vi "Measure Pulse Guard Pulse Width.vi"(7 "Pulse Phase":enum16{"Stimulus", "Recovery"}(ring), 8 "error in (no error)":errorcluster, 9 "Second Edge Threshold":dbl=4.25, 10 "First Edge Threshold":dbl=5.25, 11 "Input Waveform":waveform(dbl)={"t0"=timestamp(3473263002.422 s since 1904-01-01), "dt"=1e-05, "Y"=[]}) -> (0 "error out":errorcluster, 2 "Pulse Width":dbl)   [LabVIEW 2010]
uses:
  <vilib>/measure/mamon.llb/Waveform Peak Detection for 1 Chan.vi
  <vilib>/measure/NI_MAPro.lvlib
panel:
  out "Waveform in ( graph )":dbl[](graph)
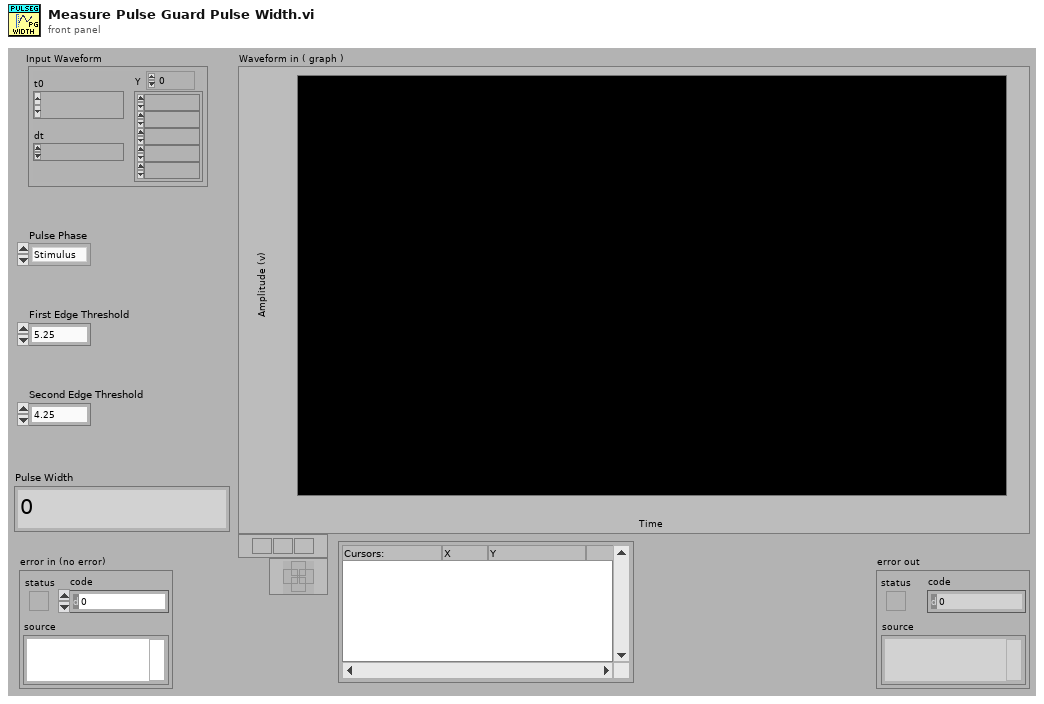
[diagram p1: front panel]
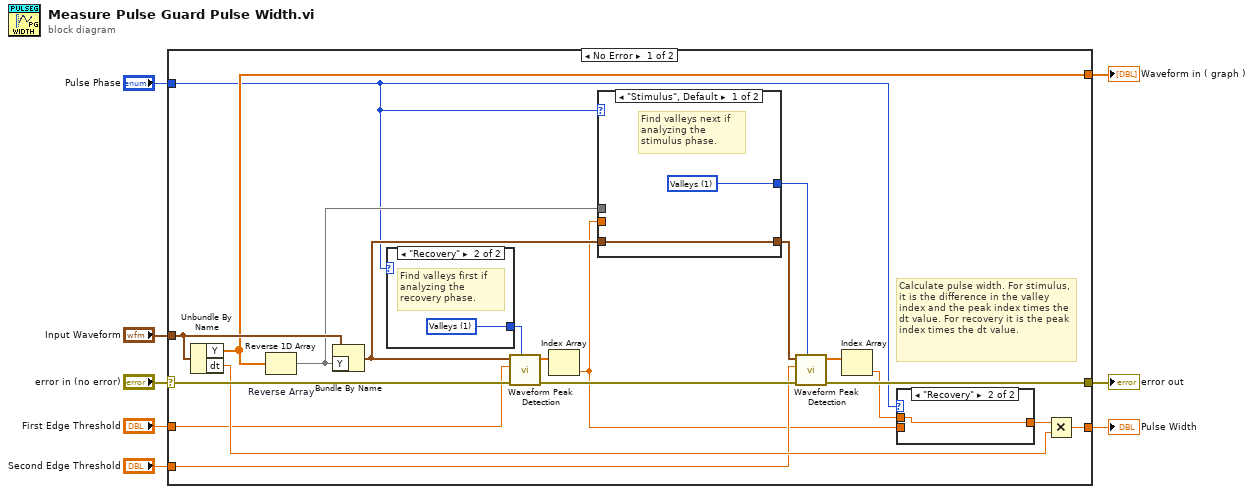
[diagram p0: block diagram]
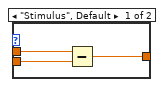
[diagram p2: hidden frame]
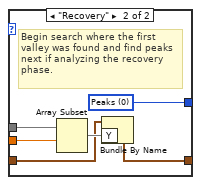
[diagram p3: hidden frame]
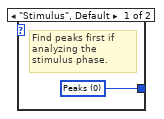
[diagram p4: hidden frame]
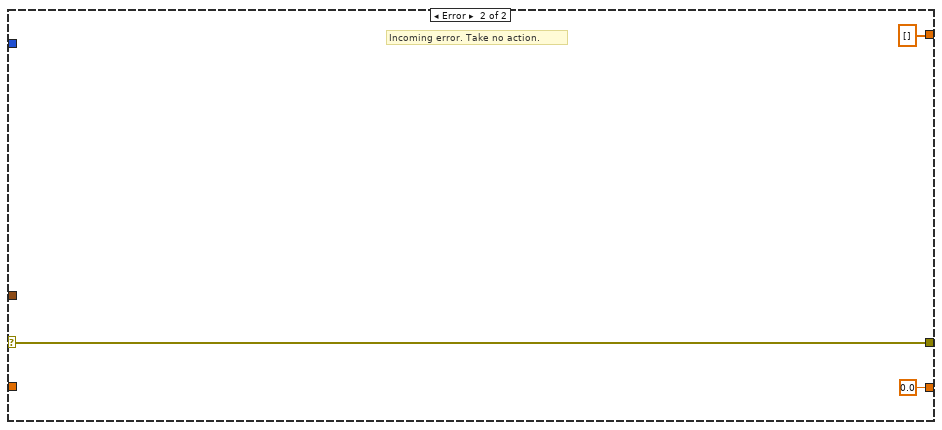
[diagram p5: hidden frame]
diagram:
  n1 = case shown="No Error" "error in (no error)" {
    selector: "error in (no error)" -> [w19 w45]
    tunnel: [w17 0.0] -> w8
    tunnel: [w18 dbl[] [] ("Y")] -> w7
    tunnel: "Second Edge Threshold" -> [w15 _]
    tunnel: "First Edge Threshold" -> [w9 _]
    tunnel: [w26 w45] -> w3
    tunnel: "Input Waveform" -> [w27 _]
    tunnel: "Pulse Phase" -> [w11 _]
    frame No Error {
      # "Calculate pulse width. For stimulus, it is the difference in the valley index and the peak index times the dt value. For recovery it is the peak index times the dt value."
      n2 = Unbundle By Name(w27) -> ("Y"=w18:dbl[], "dt"=w16:dbl)
      n3 = Reverse 1D Array "Reverse Array"(array=w18) -> (reversed array=w14:dbl[])
      n4 = Bundle By Name(cluster=w27, "Y"=w14) -> (w28:waveform(dbl))
      n5 = case shown="\"Recovery\"" w11 {
        tunnel: [w41 w42] -> w24
        frame "Stimulus", Default {
          w41 = u16 0 items=["Peaks", "Valleys"] ("peaks/valleys")
          # "Find peaks first if analyzing the stimulus phase."
        }
        frame "Recovery" {
          w42 = u16 1 items=["Peaks", "Valleys"] ("peaks/valleys")
          # "Find valleys first if analyzing the recovery phase."
        }
      }
      n6 = call-poly <vilib>:"Waveform Peak Detection.vi"("peaks/valleys"=w24, "error in"=w19, "threshold"=w9, "Signal In"=w28) -> ("error out"=w25:errorcluster, "Locations"=w23:dbl[])  [unwired: 3 in, 3 out]
      n7 = Index Array(array=w23) -> (element=w13:dbl)  [unwired: 1 in]
      n8 = case shown="\"Stimulus\", Default" w11 {
        tunnel: w14 -> [_ w40]
        tunnel: w13 -> [_ w39]
        tunnel: w28 -> [w34 w37]
        tunnel: [w34 w36] -> w12
        tunnel: [w33 w35] -> w10
        frame "Stimulus", Default {
          w33 = u16 1 items=["Peaks", "Valleys"] ("peaks/valleys")
          # "Find valleys next if analyzing the stimulus phase."
        }
        frame "Recovery" {
          w35 = u16 0 items=["Peaks", "Valleys"] ("peaks/valleys")
          # "Begin search where the first valley was found and find peaks next if analyzing the recovery phase."
          n9 = Array Subset(array=w40, index=w39) -> (w38:dbl[])  [unwired: 1 in]
          n10 = Bundle By Name(cluster=w37, "Y"=w38) -> (w36:waveform(dbl))
        }
      }
      n11 = call-poly <vilib>:"Waveform Peak Detection.vi"("peaks/valleys"=w10, "error in"=w25, "threshold"=w15, "Signal In"=w12) -> ("error out"=w26:errorcluster, "Locations"=w22:dbl[])  [unwired: 3 in, 3 out]
      n12 = Index Array(array=w22) -> (element=w21:dbl)  [unwired: 1 in]
      n13 = case shown="\"Recovery\"" w11 {
        tunnel: w21 -> [w31 w32]
        tunnel: [w30 w32] -> w20
        tunnel: w13 -> [w29 _]
        frame "Stimulus", Default {
          n14 = Subtract(x=w31, y=w29) -> (x-y=w30:dbl)
        }
        frame "Recovery" {
        }
      }
      n15 = Multiply(x=w20, y=w16) -> (x*y=w17:dbl)
    }
    frame Error {
      # "Incoming error. Take no action."
    }
  }
  "Waveform in ( graph )" <- w7
  "Pulse Width" <- w8
  "error out" <- w3
